vi "Read Boolean Assertion Type.vi"(8 "error in (no error)":errorcluster, 11 "Boolean Assertion in":refnum<class "Boolean Assertion.lvclass">) -> (0 "error out":errorcluster, 2 "Boolean Assertion Type":T1, 3 "Boolean Assertion out":refnum<class "Boolean Assertion.lvclass">)   [LabVIEW 2020, in "MacroAssert.lvlib" / "Boolean Assertion.lvclass"]
uses:
  Boolean Assertion.lvclass
  Boolean Assertion Type.ctl
  Boolean Assertion.lvclass/Boolean Assertion.ctl
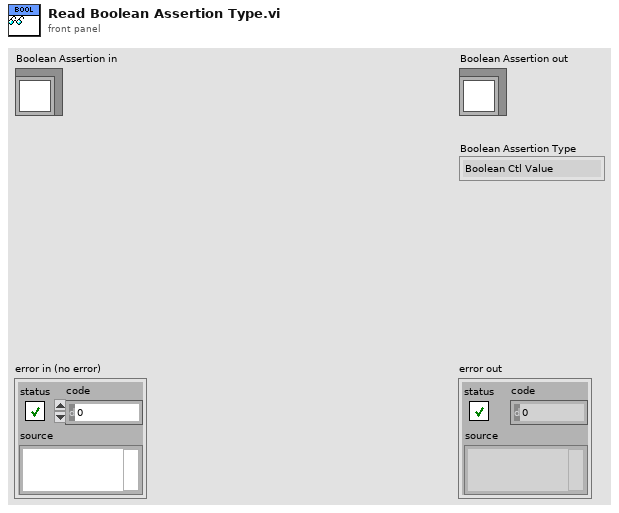
[diagram p1: front panel]
types:
  T1 = typedef "MacroAssert.lvlib/Boolean Assertion.lvclass/Boolean Assertion Type.ctl" = enum16{"Boolean Ctl Value", "Ctl Visible Property", "Ctl is Enabled", "Ctl is Grayed Out", "Ctl Key Focus Property", "Window is in Running Windows", "VI Front Panel is Open"}
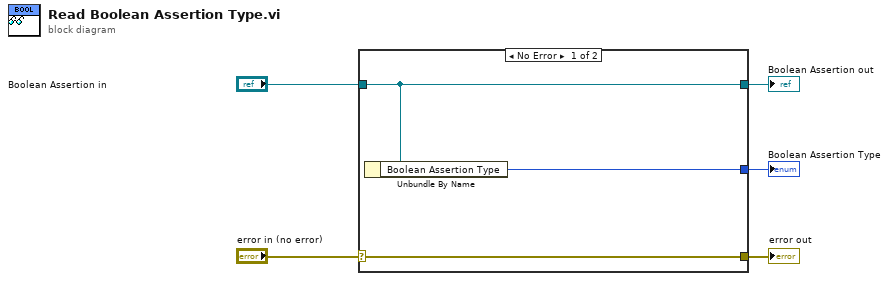
[diagram p0: block diagram]
diagram:
  n1 = case shown="No Error" "error in (no error)" {
    selector: "error in (no error)" -> [w8 w9]
    tunnel: [w8 w9] -> w4
    tunnel: [w7 w10] -> w2
    tunnel: "Boolean Assertion in" -> [w7 w10]
    tunnel: [w6 _] -> w1
    frame No Error {
      n2 = Unbundle By Name(w7) -> ("Boolean Assertion Type"=w6:T1)
    }
    frame Error {
    }
  }
  "error out" <- w4
  "Boolean Assertion out" <- w2
  "Boolean Assertion Type" <- w1
